vi "Parsed Joystick Values.vi"(8 "error in (no error)":errorcluster, 11 "JoystickDevRef":T3={"Device"=enum."USB 1"}) -> (0 "error out":errorcluster, 1 "Buttons":T1, 2 "Axes":T2, 3 "JoystickDevRef":T3={"Device"=enum."USB 1"}, 4 "POV Angle":i16)   [LabVIEW 2014]
doc: "Selects proper joystick axes / button mapping for different joysticks."
uses:
  <vilib>/Rock Robotics/WPI/Joystick/WPI_JoystickDevRef.ctl
  <vilib>/Rock Robotics/WPI/Joystick/WPI_JoystickDeviceEnum.ctl
  Typedefs/Teleop/Joystick Axes.ctl
  Typedefs/Teleop/Joystick Buttons.ctl
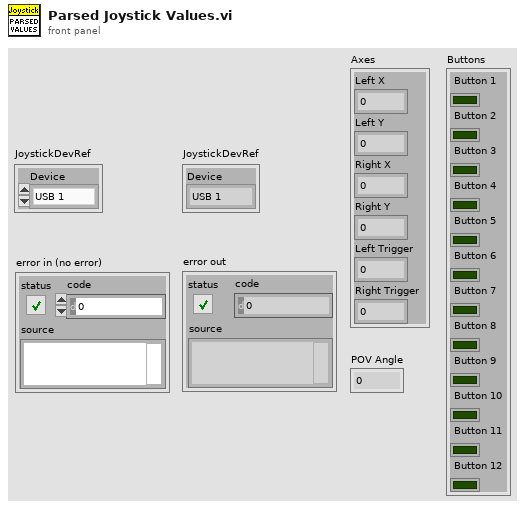
[diagram p1: front panel]
types:
  T1 = typedef "Joystick Buttons.ctl" = cluster{"Button 1":bool, "Button 2":bool, "Button 3":bool, "Button 4":bool, "Button 5":bool, "Button 6":bool, "Button 7":bool, "Button 8":bool, "Button 9":bool, "Button 10":bool, "Button 11":bool, "Button 12":bool}
  T2 = typedef "Joystick Axes.ctl" = cluster{"Left X":dbl, "Left Y":dbl, "Right X":dbl, "Right Y":dbl, "Left Trigger":dbl, "Right Trigger":dbl}
  T3 = typedef "WPI_JoystickDevRef.ctl" = cluster{"Device":T4}
  T4 = typedef "WPI_JoystickDeviceEnum.ctl" = enum16{"USB 0", "USB 1", "USB 2", "USB 3", "USB 4", "USB 5"}
  T5 = typedef "WPI_Joystick Info.ctl" = cluster{"Device Name":string, "HID Type":T6, "XBox Type":T7, "Axes Count":i32, "Axes Types":T8[], "Button Count":i32, "POV Count":i32}
  T6 = typedef "WPI_JoystickHID Types.ctl" = enum16{"Not HID", "HID Joystick", "HID Gamepad", "HID Driving Wheel", "HID Flightstick", "HID First Person"}
  T7 = typedef "WPI_JoystickXBox Types.ctl" = enum16{"Not XBox", "XBox Unknown", "XBox Gamepad", "XBox Wheel", "XBox Arcade Stick", "XBox Flight Stick", "XBox Dance Pad", "XBox Guitar", "XBox Drum Kit", "XBox Arcade Pad"}
  T8 = typedef "WPI_JoystickAxis Types.ctl" = enum16{"X Axis", "Y Axis", "Z Axis", "RxAxis", "RyAxis", "RzAxis", "Slider", "POV", "None", "L X Axis", "L Y Axis", "L Trigger", "R Trigger", "R X Axis", "R Y Axis"}
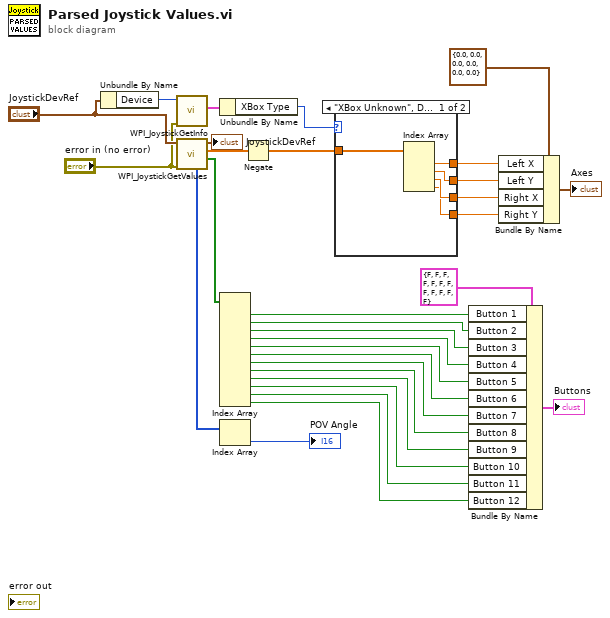
[diagram p0: block diagram]
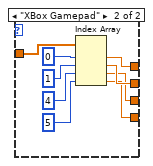
[diagram p2: hidden frame]
diagram:
  n1 = Unbundle By Name("JoystickDevRef") -> ("Device"=w31:T4)
  n2 = call <vilib>:"WPI_JoystickGetInfo.vi"("error in (no error)"="error in (no error)", "JoystickDevice"=w31) -> ("Joystick Info"=w28:T5)  [unwired: 8 in, 1 out]
  n3 = call <vilib>:"WPI_JoystickGetValues.vi"("error in (no error)"="error in (no error)", "JoystickDevRef"="JoystickDevRef") -> ("Buttons"=w14:bool[], "Axes"=w25:dbl[], "JoystickDevRef"=→"JoystickDevRef":T3, "POVs"=w16:i16[])  [unwired: 5 in, 1 out]
  n4 = Unbundle By Name(w28) -> ("XBox Type"=w27:T7)
  n5 = Index Array(array=w14) -> (element #1=w12:bool, element #2=w11:bool, element #3=w10:bool, element #4=w9:bool, element #5=w8:bool, element #6=w7:bool, element #7=w6:bool, element #8=w5:bool, element #9=w4:bool, element #10=w3:bool, element #11=w2:bool, element #12=w1:bool)  [unwired: 12 in]
  n6 = Index Array(array=w16) -> (element=→"POV Angle":i16)  [unwired: 1 in]
  n7 = Negate(x=w25) -> (-x=w13:dbl[])
  n8 = case shown="\"XBox Unknown\", Default" w27 {
    tunnel: w13 -> [w32 w45]
    tunnel: [w36 w44] -> w23
    tunnel: [w35 w43] -> w22
    tunnel: [w34 w42] -> w21
    tunnel: [w33 w41] -> w20
    frame "XBox Unknown", Default {
      n9 = Index Array(array=w32) -> (element #1=w36:dbl, element #2=w35:dbl, element #3=w34:dbl, element #4=w33:dbl)  [unwired: 4 in]
    }
    frame "XBox Gamepad" {
      n10 = Index Array(array=w45, index #1=0 ("index"), index #2=1 ("index"), index #3=4 ("index"), index #4=5 ("index")) -> (element #1=w44:dbl, element #2=w43:dbl, element #3=w42:dbl, element #4=w41:dbl)
    }
  }
  n11 = Bundle By Name(cluster=T1 {"Button 1"=FALSE, "Button 2"=FALSE, "Button 3"=FALSE, "Button 4"=FALSE, "Button 5"=FALSE, "Button 6"=FALSE, "Button 7"=FALSE, "Button 8"=FALSE, "Button 9"=FALSE, "Button 10"=FALSE, "Button 11"=FALSE, "Button 12"=FALSE} ("Joystick Buttons"), "Button 1"=w12, "Button 2"=w11, "Button 3"=w10, "Button 4"=w9, "Button 5"=w8, "Button 6"=w7, "Button 7"=w6, "Button 8"=w5, "Button 9"=w4, "Button 10"=w3, "Button 11"=w2, "Button 12"=w1) -> (→"Buttons":T1)
  n12 = Bundle By Name(cluster=T2 {"Left X"=0.0, "Left Y"=0.0, "Right X"=0.0, "Right Y"=0.0, "Left Trigger"=0.0, "Right Trigger"=0.0} ("Joystick Axes"), "Left X"=w23, "Left Y"=w22, "Right X"=w21, "Right Y"=w20) -> (→"Axes":T2)
